vi "Upgrade to Ultimate.vi"(0 "path":string) -> (4 "result":i32)   [LabVIEW 2010]
uses:
  <vilib>/Platform/browser.llb/Open URL in Default Browser (string).vi
  C:/Program Files (x86)/SoftwareKey/Instant PLUS/IP2Lib32.dll
panel:
  in  "Exit":bool
  in  "Activate":bool
  in  "Purchase":bool
  # "Autoware v2.0.0"
  # "Upgrade to Ultimate"
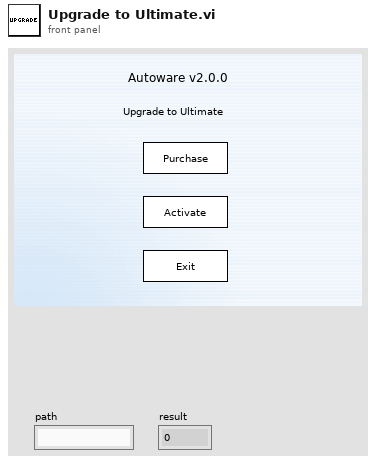
[diagram p1: front panel]
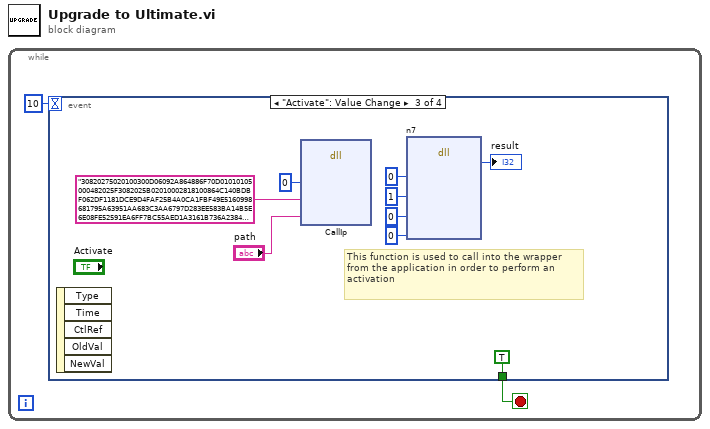
[diagram p0: block diagram]
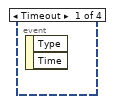
[diagram p2: hidden frame]
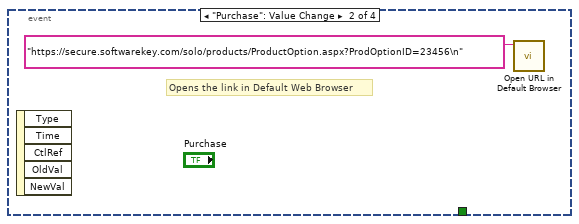
[diagram p3: hidden frame]
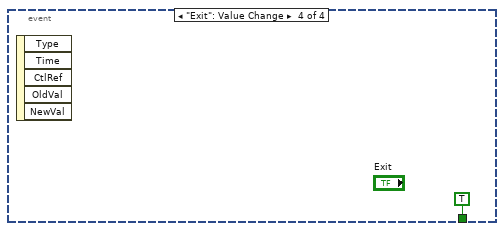
[diagram p4: hidden frame]
diagram:
  n1 = while {
    stop <- w1 stop-if-true
    n2 = event shown="[2] \"Activate\": Value Change" {
      selector: _ -> [_ _ _ _]
      dyn-events: _ -> [_ _ _ _]
      timeout: 10 -> [_ _ _ _]
      tunnel: [_ _ TRUE ("Exit") TRUE ("Exit")] -> w1
      event Timeout {
        n3 = event-data() -> ()  [unwired: 1 in, 2 out]
      }
      event "Purchase": Value Change {
        # "Opens the link in Default Web Browser"
        n4 = event-data() -> ()  [unwired: 1 in, 5 out]
        n5 = call-poly <vilib>:"Open URL in Default Browser.vi"("URL"="https://secure.softwarekey.com/solo/products/ProductOption.aspx?ProdOptionID=23456\n") -> ()  [unwired: 5 in, 2 out]
      }
      event "Activate": Value Change {
        # "This function is used to call into the wrapper from the application in order to perform an activation"
        n6 = event-data() -> ()  [unwired: 1 in, 5 out]
        n7 = dll-call lib="C:/Program Files (x86)/SoftwareKey/Instant PLUS/IP2Lib32.dll" fn="CallIp"("flags"=0, "key"="30820275020100300D06092A864886F70D01010105000482025F3082025B02010002818100864C140BDBF062DF1181DCE9D4FAF25B4A0CA1FBF49E5160998681795A63951AA683C3AA6797D283EE583BA14B5E6E08FE52591EA6FF7BC55AED1A3161B736A2384D870C7207CC8E0C44F3FA09198B5C5B93A3664E7E03A0649458AD77C39D105654BF6D9AB9740C204A6EEE81CCFF07CA72CE9B1B6C7B6A51E0E7FB828A71050201110281802B72F76D3FA09875587CD687E305E4FF6AC7DA0DC0151A53F56F48019D3E55E2F9A319A81274E239BE0D7CB42EF8E75D4338C27ADBAD02657F4CB5A6908E193403A635934E3586225F27BF45D9C9E9ED9CFCFD5F08C52C6CFB1FB7415746DD7D51C4C534D770EAAE174BC1FFC315035FFAA70DEA8A613053DEEFD2921B82A04302...", "path"="path") -> ()  [unwired: 7 in, 2 out]
        n8 = dll-call lib="C:/Program Files (x86)/SoftwareKey/Instant PLUS/IP2Lib32.dll" fn="n7"("flags"=0, "action"=1, "action_flags"=0, "handle"=0) -> ("result"=→"result":i32)  [unwired: 7 in, 2 out]
      }
      event "Exit": Value Change {
        n9 = event-data() -> ()  [unwired: 1 in, 5 out]
      }
    }
  }
